vi "DataSource Device Select.vi"(10 "Version Path":path, 11 "Data In":string[](array[string])) -> (2 "OK？":bool, 3 "Data Out":string[](array[string]))   [LabVIEW 2020]
uses:
  64c20e78-5e38-4544-a3be-bb95b41b82a3.vi
  31351a87-bfd2-4b2f-851f-df9be7303a73.vi
  <vilib>/Utility/file.llb/Read Delimited Spreadsheet (string).vi
panel:
  in  "启用？":bool
  in  "Remark":string caption="备注"
  in  "Cancle":bool
  in  "OK":bool
  in  "Device Driver":u16(ring) caption="设备驱动" items=["", "Siemens S7 Series", "Faith FT6400 Series", "ZLG_CAN", "FCTS DAQ", "Tonghui TH2600 Series", "Hioki BT3500 Series", "Yokogawa WT8500 Series", "NI_PCIE_6509", "NI_PCIE_4353_32TC", "NI_PCIE_6509_DO", "DataGraph", "TCPTransfer", "DataEmulator", "Data Forwarding Module", "NBT Test", "NBT ALIN", "Calculate_DataSource", "WarningLog", "IVCurve", "IVCurveAnalysis", "LoadControl", "FlowChart", "DataMonitor", "RHCalculate", "ControlPanel", "Data Graph", "CVM", "Device_Status", "Device_Status1", "Parameter_Set", "DataSave", "ControlPanel0", "Panel01", "SurgeTest", "GasMixtureSetting", "LinFlowChart", "Serial Port", "TCP"]
  in  "Device Model":u16(ring) caption="设备型号" items=["", "Siemens S7 Series", "Faith FT6400 Series", "ZLG_CAN", "FCTS DAQ", "Tonghui_TH2683A", "Hioki BT3500 Series", "Yokogawa WT8500 Series", "NI_PCIE_6509", "NI_PCIE_4353_32TC", "NI_PCIE_6509_DO", "DataGraph", "TCPTransfer", "DataEmulator", "Data Forwarding Module", "NBT Test", "NBT ALIN", "Calculate_DataSource", "WarningLog", "IVCurve", "IVCurveAnalysis", "LoadControl", "FlowChart", "DataMonitor", "RHCalculate", "ControlPanel", "Data Graph", "CVM", "Device_Status", "Device_Status1", "Parameter_Set", "DataSave", "ControlPanel0", "Panel01", "SurgeTest", "GasMixtureSetting", "LinFlowChart", "Serial Port", "TCP"]
  in  "Device Name":string caption="设备名称"
  in  "Port":u32 caption="端口号"
  in  "IP Address":string caption="IP地址"
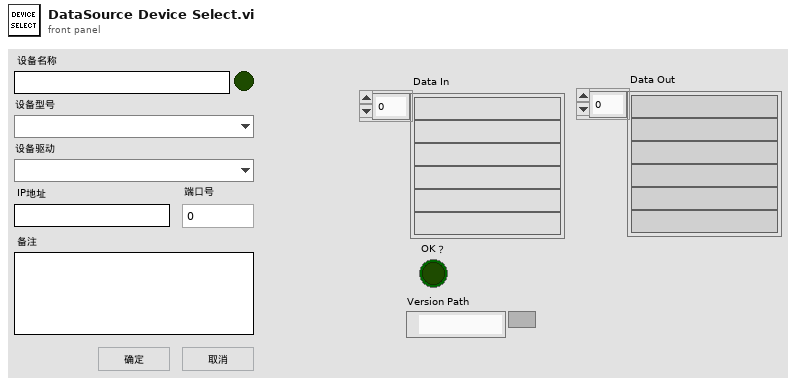
[diagram p1: front panel]
types:
  T1 = cluster{"Device Driver":string[], "Device Model":string[], "OK？":bool, "Timeout":i32, "Data In":string[]}
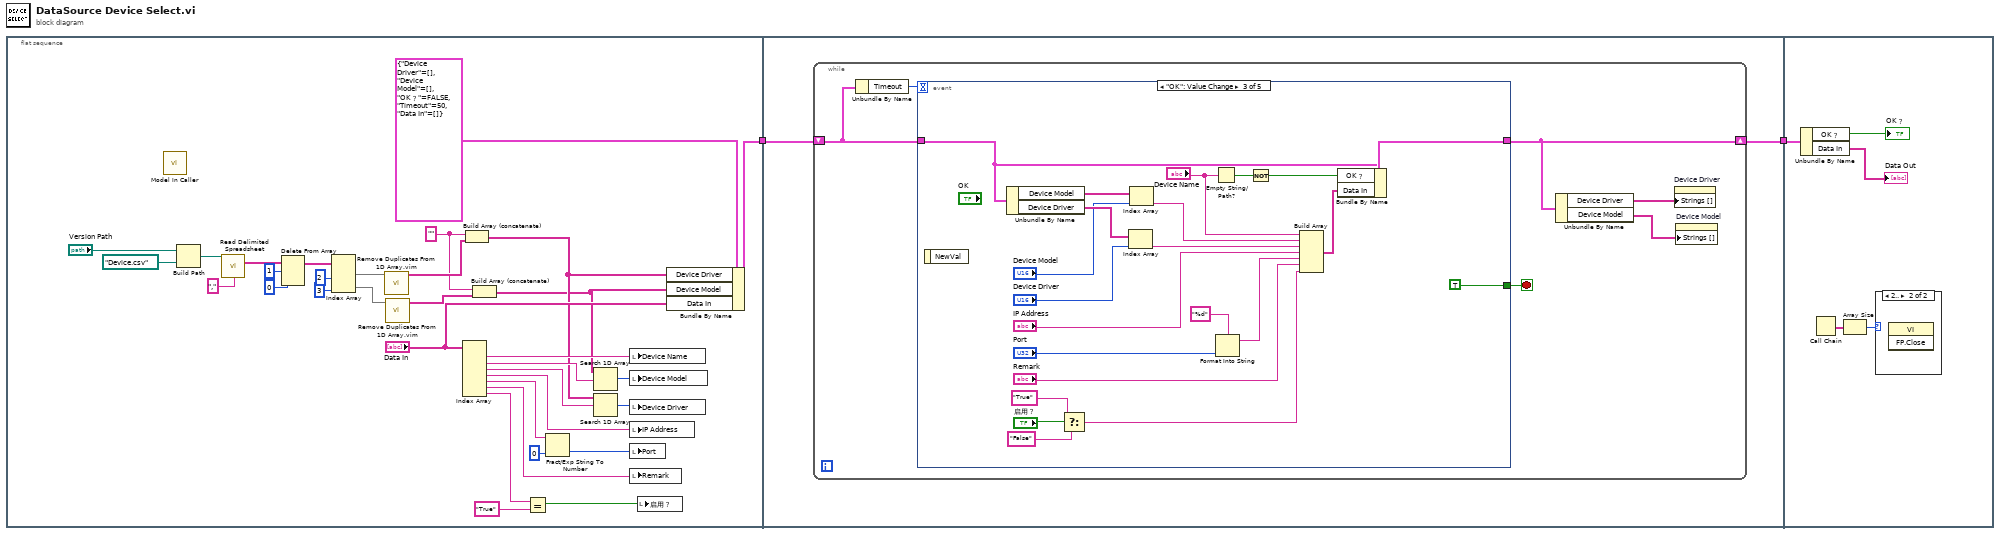
[diagram p0: block diagram]
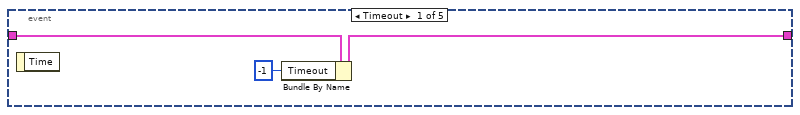
[diagram p2: hidden frame]
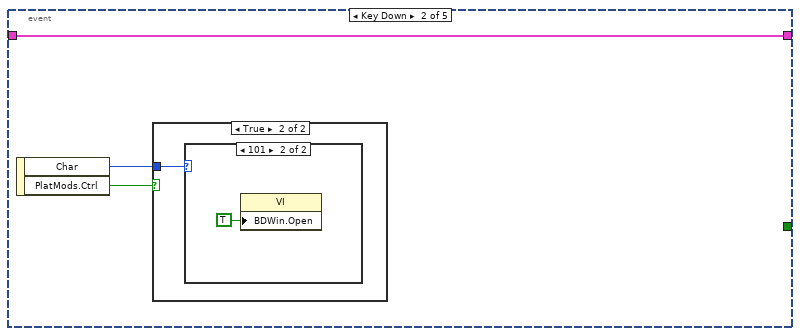
[diagram p3: hidden frame]
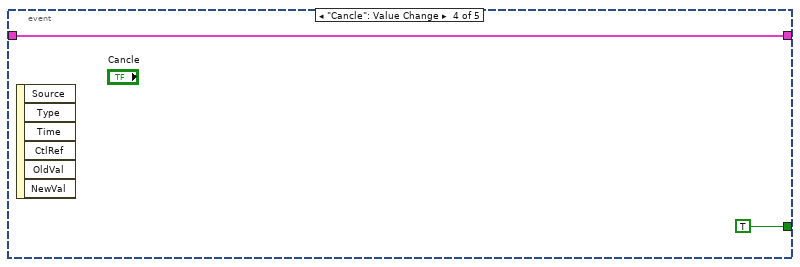
[diagram p6: hidden frame]
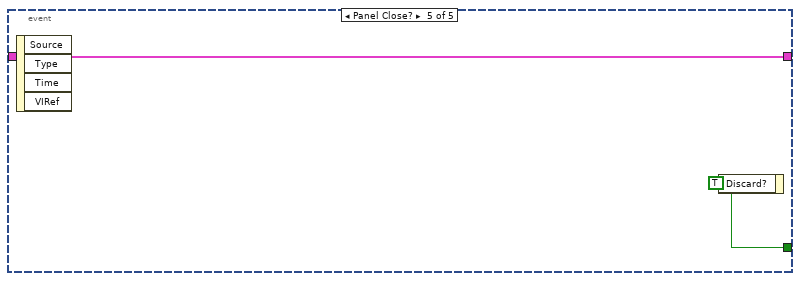
[diagram p7: hidden frame]
diagram:
  n1 = flat-sequence {
    tunnel: [w25] -> w1
    tunnel: [w37] -> w2
    tunnel: w1 -> [w36]
    tunnel: w2 -> [w80]
    frame #0 {
      w10 = ""
      n2 = call "Model In Caller.vi"() -> ()  [unwired: 11 in, 1 out]
      n3 = Build Path(base path="Version Path", name or relative path=path "Device.csv" ("名称或相对路径")) -> (appended path=w4:path)
      n4 = call-poly <vilib>:"Read Delimited Spreadsheet.vi"("file path (dialog if empty)"=w4, "delimiter (\\t)"="," ("delimiter (\\t)")) -> ("all rows"=w34:string[][])  [unwired: 8 in, 5 out]
      n5 = Delete From Array(array=w34, length=1 ("长度"), index (row)=0 ("索引 (行)")) -> (array with subset deleted=w31:string[][])  [unwired: 1 in, 1 out]
      n6 = Index Array(array=w31, index (col) #1=2 ("禁用的索引 (列)"), index (col) #2=3 ("索引 (列)")) -> (element #1=w28:string[], element #2=w27:string[])  [unwired: 2 in]
      n7 = call "Remove Duplicates From 1D Array.vim"("array"=w28) -> ("array with duplicates removed"=w13:string[])  [unwired: 10 in]
      n8 = call "Remove Duplicates From 1D Array.vim"("array"=w27) -> ("array with duplicates removed"=w11:string[])  [unwired: 10 in]
      n9 = Index Array(array="Data In") -> (element #1=w23:string, element #2=w22:string, element #3=w20:string, element #4=w18:string, element #5=w17:string, element #6=w14:string, element #7=w8:string)  [unwired: 7 in]
      n10 = Build Array (concatenate)(w10, w13) -> (w12:string[])
      n11 = Build Array (concatenate)(w10, w11) -> (w9:string[])
      n12 = Equal?(x=w8, y="True") -> (x = y?=w6:bool)
      n13 = Fract/Exp String To Number(string=w17, default (0 dbl)=u32 0 ("默认(0 DBL)")) -> (number=w15:u32)  [unwired: 2 in, 1 out]
      n14 = Search 1D Array(1D array=w9, element=w22) -> (index of element=w21:i32)  [unwired: 1 in]
      n15 = Search 1D Array(1D array=w12, element=w20) -> (index of element=w19:i32)  [unwired: 1 in]
      n16 = local write "Device Name"(w23) -> ()
      n17 = local write "Device Model"(w21) -> ()
      n18 = local write "Device Driver"(w19) -> ()
      n19 = local write "IP Address"(w18) -> ()
      n20 = local write "Port"(w15) -> ()
      n21 = local write "Remark"(w14) -> ()
      n22 = local write "启用？"(w6) -> ()
      n23 = Bundle By Name(cluster=T1 {"Device Driver"=[], "Device Model"=[], "OK？"=FALSE, "Timeout"=50, "Data In"=[]}, "Device Driver"=w12, "Device Model"=w9, "Data In"="Data In") -> (w25:T1)
    }
    frame #1 {
      n24 = while {
        shift-right: [w42] -> w37
        shift-left: w36 -> [w39]
        stop <- w43 stop-if-true
        n25 = Unbundle By Name(w39) -> ("Timeout"=w38:i32)
        n26 = event shown="[2] \"OK\": Value Change" {
          selector: _ -> [_ _ _ _ _]
          dyn-events: _ -> [_ _ _ _ _]
          timeout: w38 -> [_ _ _ _ _]
          tunnel: [_ _ TRUE ("放弃？") TRUE ("放弃？") w77] -> w43
          tunnel: [w45 w47 w72 w74 w76] -> w42
          tunnel: w39 -> [w46 w47 w69 w74 w76]
          event Timeout {
            n27 = event-data() -> ()  [unwired: 1 in, 1 out]
            n28 = Bundle By Name(cluster=w46, "Timeout"=-1) -> (w45:T1)
          }
          event Key Down {
            n29 = event-data() -> ("Char"=w49:i16, "PlatMods.Ctrl"=w48:bool)  [unwired: 1 in]
            n30 = case shown="True" w48 {
              tunnel: w49 -> [_ w50]
              frame False {
              }
              frame True {
                n31 = case shown="101" w50 {
                  frame 0, Default {
                  }
                  frame 101 {
                    n32 = property class="VI"("BDWin.Open"=TRUE ("程序框图窗口:打开")) -> ()  [unwired: 2 in, 2 out]
                  }
                }
              }
            }
          }
          event "OK": Value Change {
            n33 = event-data() -> ()  [unwired: 1 in, 1 out]
            n34 = Unbundle By Name(w69) -> ("Device Model"=w68:string[], "Device Driver"=w65:string[])
            n35 = Select(t="True" ("y"), s="启用？", f="False" ("y")) -> (s? t:f=w52:string)
            n36 = Index Array(array=w65, index="Device Driver") -> (element=w62:string)
            n37 = Index Array(array=w68, index="Device Model") -> (element=w66:string)
            n38 = Empty String/Path?(string/path="Device Name") -> (empty?=w71:bool)
            n39 = Format Into String(format string="%d" ("格式字符串"), "Port") -> (resulting string=w58:string)  [unwired: 2 in, 1 out]
            n40 = Not(x=w71) -> (.not. x?=w70:bool)
            n41 = Build Array("Device Name", w66, w62, "IP Address", w58, "Remark", w52) -> (w57:string[])
            n42 = Bundle By Name(cluster=w69, "OK？"=w70, "Data In"=w57) -> (w72:T1)
          }
          event "Cancle": Value Change {
            n43 = event-data() -> ()  [unwired: 1 in, 6 out]
          }
          event Panel Close? {
            w77 = TRUE ("放弃？")
            n44 = event-data() -> ()  [unwired: 1 in, 4 out]
            n45 = event-data("Discard?"=w77) -> ()  [unwired: 1 in, 1 out]
          }
        }
        n46 = Unbundle By Name(w42) -> ("Device Driver"=w41:string[], "Device Model"=w40:string[])
        n47 = property on="Device Driver" class="Ring (严格)"("Strings []"=w41) -> ()  [unwired: 2 in, 2 out]
        n48 = property on="Device Model" class="Ring (严格)"("Strings []"=w40) -> ()  [unwired: 2 in, 2 out]
      }
    }
    frame #2 {
      n49 = Unbundle By Name(w80) -> ("OK？"=→"OK？":bool, "Data In"=→"Data Out":string[])
      n50 = Call Chain() -> (call chain=w82:string[])
      n51 = Array Size(array=w82) -> (size(s)=w81:i32)
      n52 = case shown="2.." w81 {
        frame 0, Default {
        }
        frame 2.. {
          n53 = invoke class="VI" method="FP.Close"() -> ()  [unwired: 3 in, 3 out]
        }
      }
    }
  }
